vi "FrameCmdB.vi"(8 "error in":errorcluster, 10 "DataMessage":T1={"Send Debug"="", "idx"=0, "DataType"=enum."Int", "Cmd id"=200, "Get/Set"=enum."Set"}) -> (0 "error out":errorcluster, 1 "Get/Set":enum8{"Set", "Get"}(ring), 2 "output array":u8[](array[numeric]) format="%.0x", 3 "DataToSend":string)   [LabVIEW 2017]
uses:
  data/Crc16DLL.dll
panel:
  out "CRCout":u16 format="%.0x"
  # "2882400010"
  # "Value"
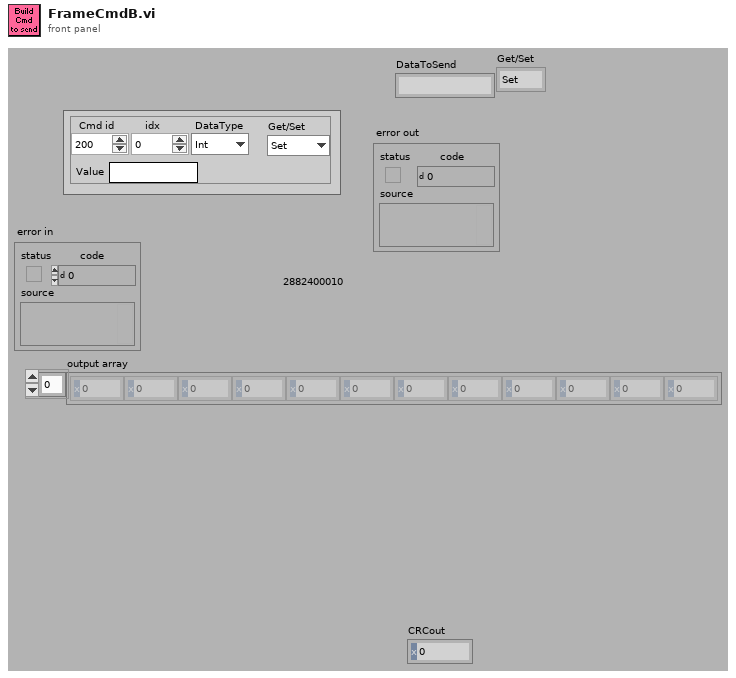
[diagram p1: front panel]
types:
  T1 = cluster{"Send Debug":string, "idx":u16, "DataType":enum8{"Int", " float"}, "Cmd id":u16, "Get/Set":enum8{"Set", "Get"}}
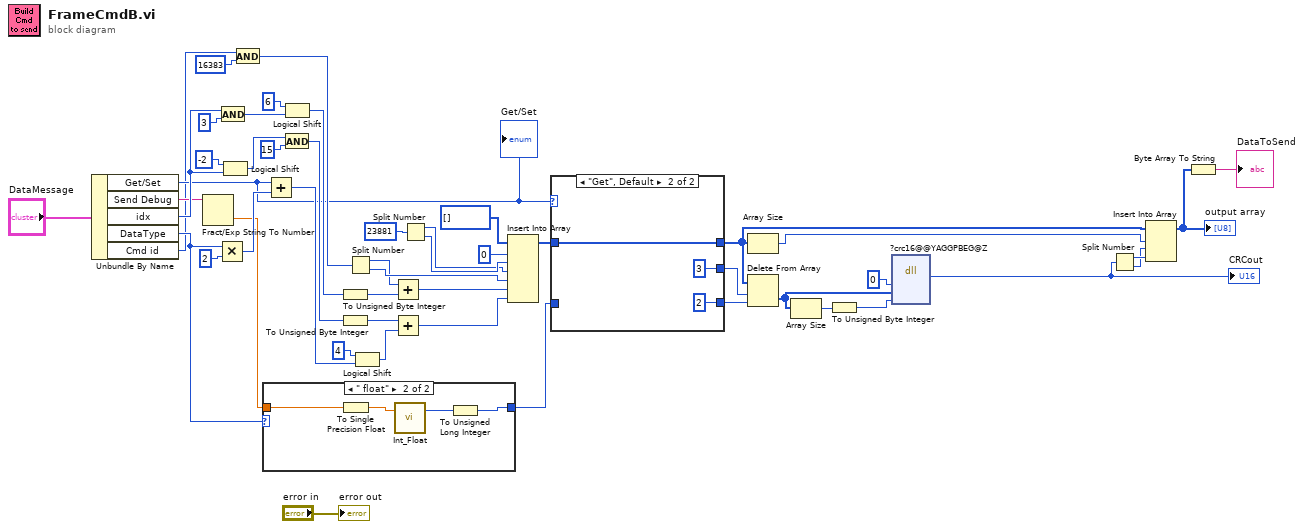
[diagram p0: block diagram]
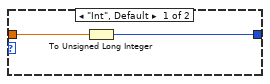
[diagram p2: hidden frame]
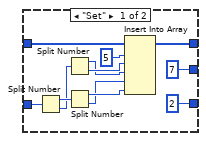
[diagram p3: hidden frame]
diagram:
  n1 = Unbundle By Name("DataMessage") -> ("Get/Set"=w3:enum8{"Set", "Get"}, "Send Debug"=w6:string, "idx"=w8:u16, "DataType"=w2:enum8{"Int", " float"}, "Cmd id"=w1:u16)
  "Get/Set" <- w3
  n2 = Fract/Exp String To Number(string=w6) -> (number=w7:dbl)  [unwired: 3 in, 1 out]
  n3 = Multiply(x=w2, y=u8 2) -> (x*y=w41:u8)
  n4 = And(x=w8, y=u16 3) -> (x .and. y?=w25:u16)
  n5 = Logical Shift(y=i16 -2, x=w8) -> (x << y=w35:u16)
  n6 = And(x=w1, y=u16 16383) -> (x .and. y?=w29:u16)
  n7 = case shown="\" float\"" w2 {
    tunnel: [w50 w53] -> w5
    tunnel: w7 -> [w51 w52]
    frame "Int", Default {
      n8 = To Unsigned Long Integer(number=w51) -> (unsigned 32bit integer=w50:u32)
    }
    frame " float" {
      n9 = To Single Precision Float(number=w52) -> (single precision float=w55:sgl)
      n10 = call "Int_Float.vi"("1 Float in"=w55) -> ("1 Int out"=w54:i32)  [unwired: 1 in, 1 out]
      n11 = To Unsigned Long Integer(number=w54) -> (unsigned 32bit integer=w53:u32)
    }
  }
  n12 = Add(x=w3, y=w41) -> (x+y=w39:u8)
  n13 = Logical Shift(y=i16 6, x=w25) -> (x << y=w24:u16)
  n14 = And(x=w35, y=u16 15) -> (x .and. y?=w32:u16)
  n15 = To Unsigned Byte Integer(number=w24) -> (unsigned 8bit integer=w26:u8)
  n16 = To Unsigned Byte Integer(number=w32) -> (unsigned 8bit integer=w30:u8)
  n17 = Split Number(x=w29) -> (hi(x)=w28:u8, lo(x)=w44:u8)
  n18 = Logical Shift(y=i8 4, x=w39) -> (x << y=w33:u8)
  n19 = Add(x=w28, y=w26) -> (x+y=w27:u8)
  n20 = Add(x=w30, y=w33) -> (x+y=w31:u8)
  n21 = Split Number(x=u16 23881 ("MagicNumber")) -> (hi(x)=w46:u8, lo(x)=w47:u8)
  n22 = Insert Into Array(array=u8[] [] ("array_in"), index=0, new element #1=w47, new element #2=w46, new element #3=w44, new element #4=w27, new element #5=w31) -> (w22:u8[])
  n23 = case shown="\"Get\", Default" w3 {
    tunnel: w22 -> [w67 w70]
    tunnel: [w66 w70] -> w21
    tunnel: [7 ("length") 3 ("length")] -> w20
    tunnel: [2 ("index") 2 ("index")] -> w19
    tunnel: w5 -> [w56 _]
    frame "Set" {
      n24 = Split Number(x=w56) -> (hi(x)=w63:u16, lo(x)=w62:u16)
      n25 = Split Number(x=w62) -> (hi(x)=w60:u8, lo(x)=w61:u8)
      n26 = Split Number(x=w63) -> (hi(x)=w59:u8, lo(x)=w58:u8)
      n27 = Insert Into Array(array=w67, index=5, new element #1=w61, new element #2=w60, new element #3=w58, new element #4=w59) -> (w66:u8[])
    }
    frame "Get", Default {
    }
  }
  n28 = Array Size(array=w21) -> (size(s)=w13:i32)
  n29 = Delete From Array(array=w21, length=w20, index=w19) -> (deleted portion=w11:u8[])  [unwired: 1 out]
  n30 = Array Size(array=w11) -> (size(s)=w12:i32)
  n31 = To Unsigned Byte Integer(number=w12) -> (unsigned 8bit integer=w18:u8)
  n32 = dll-call lib="C:/Projects/SingleBoard/LabVIEW/BurnProjet/data/Crc16DLL.dll" fn="?crc16@@YAGGPBEG@Z"("CRC"=u16 0, "buffer"=w11, "len"=w18) -> ("return type"=w16:u16)  [unwired: 6 in, 2 out]
  "CRCout" <- w16
  n33 = Split Number(x=w16) -> (hi(x)=w15:u8, lo(x)=w14:u8)
  n34 = Insert Into Array(array=w21, index=w13, new element #1=w14, new element #2=w15) -> (w10:u8[])
  "output array" <- w10
  n35 = Byte Array To String(unsigned byte array=w10) -> (string=→"DataToSend":string)
  "error out" <- "error in"
